vi "Open Report File.vi"(8 "error in (no error)":errorcluster, 11 "XML Report In":refnum<class "XML Report.lvclass">) -> (0 "error out":errorcluster, 3 "XML Report Out":refnum<class "XML Report.lvclass">)   [LabVIEW 2020, in "XML Report.lvclass"]
uses:
  XML Report.lvclass
  Core/Result/Result.ctl
  Core/Result/Status.ctl
  Core/Result/Type.ctl
  XML Report.lvclass/XML Report.ctl
  <vilib>/xml/NI_XML.lvlib
  <resource>/objmgr/DOMUserDefRef.rc
  Core/Result/Result.lvlib
  User Interface/Support/Paths.lvlib
  Framework/Report Plugin/Report Plugin.lvclass
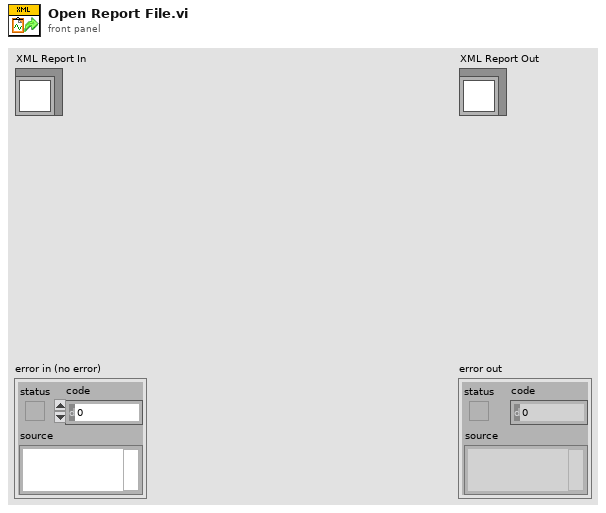
[diagram p1: front panel]
types:
  T1 = typedef "Result.lvlib/Result.ctl" = cluster{"Name":string, "Description":string, "Status":T2, "Result Type":T3, "Execution Time":dbl, "Data":cluster{"Expected":variant, "Actual":variant, "Delta":variant}}
  T2 = typedef "Result.lvlib/Status.ctl" = enum16{"", "Passed", "Failed", "Error", "Skipped", "Setup Error", "Broken", "Teardown Error"}
  T3 = typedef "Result.lvlib/Type.ctl" = enum16{"Test Case", "Test Suite", "Test Run", "Pass", "Fail", "Skip", "Pass if", "Fail if", "Pass if Error", "Fail if Error", "Pass if Equal", "Fail if Equal"}
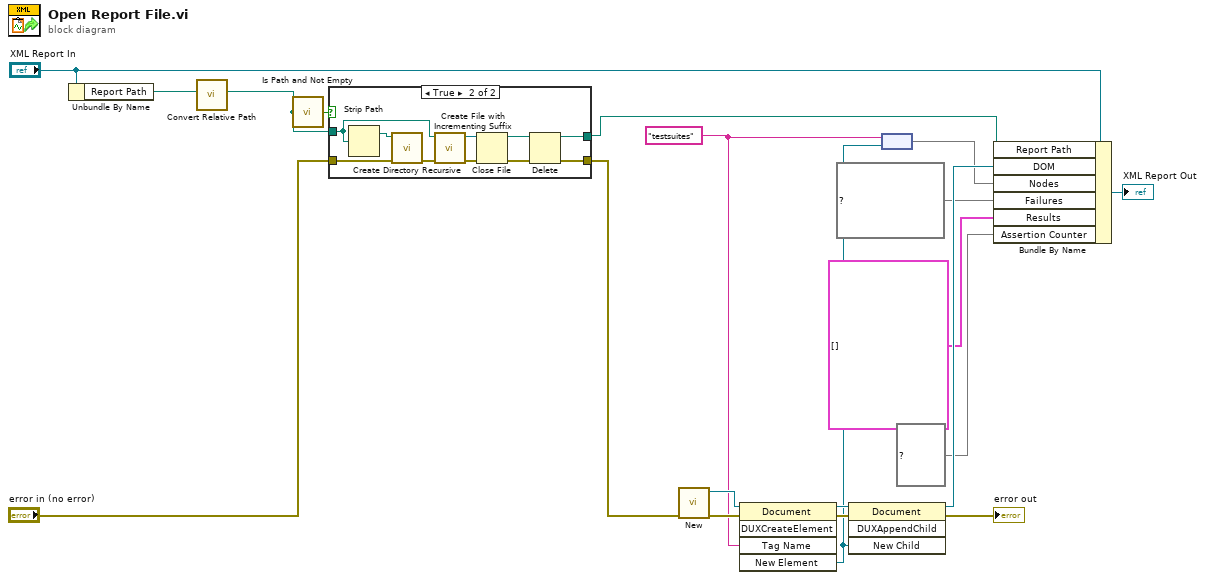
[diagram p0: block diagram]
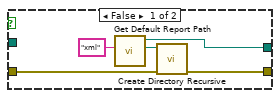
[diagram p2: hidden frame]
diagram:
  w13 = "testsuites" ("Tag Name")
  n1 = Unbundle By Name("XML Report In") -> ("Report Path"=w2:path)
  n2 = call "Convert Relative Path.vi"("File Path in"=w2) -> ("Modified Path"=w1:path)  [unwired: 10 in]
  n3 = call <vilib>:"Is Path and Not Empty.vi"("path"=w1) -> ("Is Path and Not Empty?"=w7:bool)  [unwired: 4 in]
  n4 = case shown="True" w7 {
    tunnel: w1 -> [_ w32]
    tunnel: [w25 w28] -> w4
    tunnel: "error in (no error)" -> [w24 w29]
    tunnel: [w23 w26] -> w3
    frame False {
      n5 = call "Get Default Report Path.vi"("File Extension"="xml") -> ("Default Report Directory"=w22:path, "Default Report Path"=w23:path)  [unwired: 9 in]
      n6 = call <vilib>:"Create Directory Recursive.vi"("error in (no error)"=w24, "directory"=w22) -> ("error out"=w25:errorcluster)  [unwired: 3 in, 2 out]
    }
    frame True {
      n7 = Strip Path(path=w32) -> (stripped path=w31:path)  [unwired: 1 out]
      n8 = call <vilib>:"Create Directory Recursive.vi"("error in (no error)"=w29, "directory"=w31) -> ("error out"=w30:errorcluster)  [unwired: 3 in, 2 out]
      n9 = call <vilib>:"Create File with Incrementing Suffix.vi"("error in (no error)"=w30, "file path"=w32) -> ("error out"=w33:errorcluster, "refnum out"=w34:refnum<file>)  [unwired: 7 in, 1 out]
      n10 = Close File(refnum=w34, error in=w33) -> (path=w27:path, error out=w35:errorcluster)
      n11 = Delete(path (use dialog)=w27, error in=w35) -> (deleted path=w26:path, error out=w28:errorcluster)  [unwired: 3 in, 1 out]
    }
  }
  n12 = call <vilib>:"New.vi"("error in (no error)"=w4) -> ("error out"=w16:errorcluster, "DOM document out"=w19:refnum<k20>)  [unwired: 7 in]
  n13 = invoke class="Document" method="DUXCreateElement"(reference=w19, error in=w16, "Tag Name"=w13) -> (reference out=w18:refnum<k20>, error out=w17:errorcluster, "New Element"=w12:refnum<k20>)  [unwired: 2 in, 2 out]
  n14 = invoke class="Document" method="DUXAppendChild"(reference=w18, error in=w17, "New Child"=w12) -> (reference out=w14:refnum<k20>, error out=→"error out":errorcluster)  [unwired: 1 in, 2 out]
  n15 = node(w13, w12) -> (w11:map{string, refnum<k20>})
  n16 = Bundle By Name(cluster="XML Report In", "Report Path"=w3, "DOM"=w14, "Nodes"=w11, "Failures"=map{string, refnum<k20>[]} {}, "Results"=T1[] [], "Assertion Counter"=map{string, i32} {}) -> (→"XML Report Out":refnum<class "XML Report.lvclass">)
